vi "verify if file exists.vi"(8 "error in (no error)":errorcluster, 11 "Log File in":refnum<class "Log File.lvclass">) -> (0 "error out":errorcluster, 3 "Log File out":refnum<class "Log File.lvclass">)   [LabVIEW 2018, in "Log File.lvclass"]
uses:
  Log File.lvclass
  Log File.lvclass/Log File.ctl
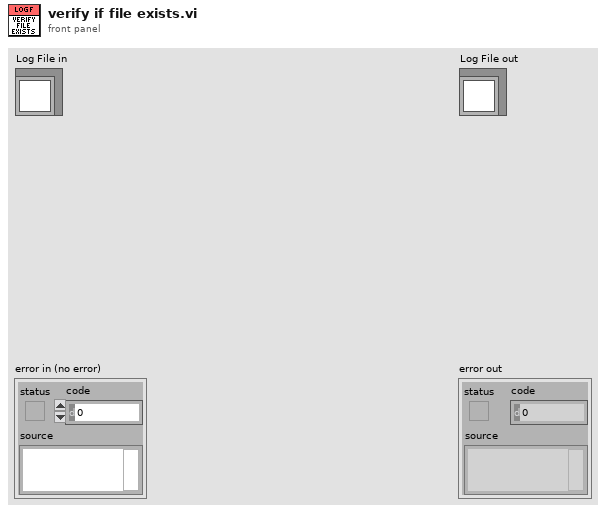
[diagram p1: front panel]
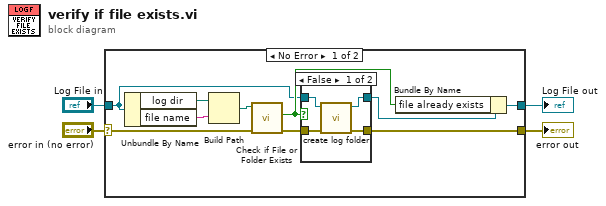
[diagram p0: block diagram]
diagram:
  n1 = case shown="No Error" "error in (no error)" {
    selector: "error in (no error)" -> [w14 w22]
    tunnel: [w5 w22] -> w3
    tunnel: [w10 w21] -> w1
    tunnel: "Log File in" -> [w8 w21]
    frame No Error {
      n2 = Unbundle By Name(w8) -> ("log dir"=w13:path, "file name"=w12:string)
      n3 = Build Path(base path=w13, name or relative path=w12) -> (appended path=w11:path)
      n4 = call <vilib>:"Check if File or Folder Exists.vi"("error in (no error)"=w14, "path"=w11) -> ("error out"=w6:errorcluster, "file or folder exists?"=w9:bool)  [unwired: 7 in, 1 out]
      n5 = case shown="False" w9 {
        tunnel: w8 -> [w18 w20]
        tunnel: [w17 w20] -> w7
        tunnel: w6 -> [w16 w19]
        tunnel: [w15 w19] -> w5
        frame False {
          n6 = call "create log folder.vi"("error in (no error)"=w16, "Log File in"=w18) -> ("error out"=w15:errorcluster, "Log File out"=w17:refnum<class "Log File.lvclass">)  [unwired: 8 in]
        }
        frame True {
        }
      }
      n7 = Bundle By Name(cluster=w7, "file already exists"=w9) -> (w10:refnum<class "Log File.lvclass">)
    }
    frame Error {
    }
  }
  "error out" <- w3
  "Log File out" <- w1
